vi "TDC_DAQV31_Paralled_muon.vi"(7 "address":string[](array[string])=["192.168.10.20"], 8 "error in (no error)":errorcluster, 9 "stop":bool, 10 "save data":bool=TRUE, 11 "SMA mode":bool=TRUE) -> (0 "error out 3":errorcluster, 2 "csv path":path=path "G:/tdc/2017/data/test_20250313_082908.csv", 3 "rate":dbl)   [LabVIEW 2017]
uses:
  gloabal.vi
  <vilib>/Utility/file.llb/Write Delimited Spreadsheet (DBL).vi
  <vilib>/Utility/file.llb/Write Delimited Spreadsheet (I64).vi
panel:
  out "x .and. y?":u64
  out "pmt trigger rate":u32[](array[numeric])
  out "event":u32[](array[numeric])
  in  "calib_file":path=path "G:/tdc/2017/data/test_20250313_032748_codeDensity.csv" caption="文件路径 （空时为对话框）"
  in  "use_calib_file":bool
  out "cal 3":u32[](graph)=[0, 0, 0, 0, 0, 0, 0, 0, 0, 0, 0, 0, 0, 0, 0, 0, 0, 0, 0, 0, 0, 0, 0, 0, 0, 0, 0, 0, 0, 0, 0, 0, 0, 0, 0, 0, 0, 0, 0, 0, 0, 0, 0, 0, 0, 0, 0, 0, 0, 0, 0, 0, 0, 0, 0, 0, 0, 0, 0, 0, 0, 0, 0, 0, 0, 0, 0, 0, 0, 0, 0, 0, 0, 0, 0, 0, 0, 0, 0, 0, 0, 0, 0, 0, 0, 0, 0, 0, 0, 0, 0, 0, 0, 0, 0, 0, 0, 0, 0, 0, 0, 0, 0, 0, 0, 0, 0, 0, 0, 0, 0, 0, 0, 0, 0, 0, 0, 0, 0, 0, 0, 0, 0, 0, 0, 0, 0, 0, 0, 0, 0, 0, 0, 0, 0, 0, 0, 0, 0, 0, 0, 0, 0, 0, 0, 0, 0, 0, 0, 0, 0, 0, 0, 0, 0, 0, 0, 0, 0, 0, 0, 0, 0, 0, 0, 15, 3, 1, 14, 3, 31, 20, 16, 6, 1, 18, 12, 4, 29, 10, 8, 29, 2, 14, 4, 25, 7, 24, 4, 0, 1, 5, 8, 18, 22, 0, 4, 5, 0, 12, 9, 9, 20, 21, 4, 10, 13, 5, 21, 13, 14, 2, 6, 13, 1, 3, 5, 10, 20, 2, 3, 4, 3, 4, 2, 20, 13, 2, 5, 1, 3, 12, 4, 1, 14, 7, 5, 4, 1, 10, 2, 21, 14, 2, 5, 10, 4, 0, 11, 19, 6, 4, 1, 37, 1, 4, 2, 1, 10, 13, 4, 8, 10, 6, 9, 2, 0, 6, 8, 12, 3, 21, 5, 7, 8, 2, 3, 7, 17, 6, 5, 6, 4, 6, 0, 2, 1, 3, 10, 33, 7, 2, 6, 3, 7, 3, 2, 0, 12, 10, 11, 13, 13, 7, 3, 9, 6, 16, 0, 13, 5, 6, 3, 0, 5, 5, 7, 1, 10, 7, 13, 14, 5, 1, 12, 7, 1, 10, 2, 1, 14, 18, 13, 11, 4, 6, 9, 22, 11, 9, 2, 2, 8, 14, 4, 4, 6, 12, 13, 3, 9, 5, 5, 1, 5, 11, 18, 3, 0, 5, 4, 6, 7, 6, 1, 13, 5, 1, 2, 2, 1, 4, 12, 7, 3, 2, 3, 9, 11, 1, 20, 3, 4, 5, 5, 3, 5, 8, 5, 3, 26, 14, 6, 1, 3, 12, 12, 4, 23, 10, 3, 4, 4, 10, 3, 5, 4, 2, 14, 5, 15, 20, 1, 5, 1, 20, 6, 1, 3, 13, 21, 12, 7, 4, 1, 5, 30, 11, 2, 4, 0, 12, 7, 10, 3, 2, 25, 6, 1, 3, 6, 3, 8, 37, 4, 6, 2, 2, 4, 3, 5, 6, 13, 6, 9, 22, 1, 3, 7, 7, 4, 8, 33, 2, 1, 15, 3, 8, 23, 21, 2, 2, 27, 13, 3, 5, 10, 4, 18, 5, 5, 8, 0, 1, 8, 12, 4, 3, 0, 4, 8, 4, 7, 4, 2, 11, 13, 3, 0, 7, 5, 3, 4, 8, 4, 20, 2, 13, 4, 8, 6, 17, 4, 2, 1, 15, 2, 15, 5, 19, 0, 4, 15, 4, 16, 11, 1, 16, 4, 6, 6, 5, 7, 3, 9, 15, 3, 6, 3, 13, 5, 7, 3, 27, 2, 0, 21, 1, 4, 1, 4, 5, 3, 10, 7, 3, 6, 4, 18, 21, 7, 6, 7, 7, 12, 6, 9, 8, 11, 12, 13, 2, 2, 5, 4, 7, 52, 3, 5, 8, 7, 10, 4, 4, 6, 5, 18, 0, 3, 6, 1, 9, 5, 19, 13, 24, 12, 4, 4, 15, 6, 41, 3, 8, 5, 17, 26, 8, 7, 20, 2, 5, 12, 10, 10, 12, 9, 17, 6, 3, 1, 5, 3, 7, 8, 4, 10, 5, 10, 7, 1, 2, 14, 7, 25, 3, 0, 0, 0, 5, 21, 8, 14, 4, 10, 2, 3, 2, 4, 8, 12, 3, 6, 8, 3, 4, 3, 20, 5, 6, 7, 8, 11, 2, 8, 6, 5, 15, 17, 10, 10, 3, 3, 9, 18, 7, 7, 3, 5, 5, 5, 2, 2, 2, 4, 1, 0, 42, 3, 14, 4, 3, 5, 2, 7, 4, 2, 7, 5, 22, 4, 3, 17, 3, 5, 8, 19, 7, 5, 0, 3, 4, 10, 1, 8, 2, 2, 13, 23, 4, 9, 5, 0, 0, 0, 27, 2, 16, 11, 15, 3, 0, 18, 2, 8, 29, 19, 6, 7, 2, 6, 12, 1, 13, 2, 7, 5, 11, 8, 5, 6, 6, 19, 2, 4, 0, 7, 22, 13, 3, 7, 3, 8, 11, 0, 3, 26, 6, 5, 5, 6, 4, 10, 17, 16, 4, 3, 4, 3, 4, 21, 8, 10, 10, 7, 0, 9, 9, 2, 10, 10, 2, 9, 9, 4, 14, 5, 5, 4, 18, 6, 3, 0, 4, 1, 20, 2, 33, 4, 1, 2, 1, 20, 6, 3, 11, 10, 2, 1, 13, 9, 6, 1, 0, 0, 0, 0, 0, 0, 0, 0, 0, 0, 0, 0, 0, 0, 0, 0, 0, 0, 0, 0, 0, 0, 0, 0, 0, 0, 0, 0, 0, 0, 0, 0, 0, 0, 0, 0, 0, 0, 0, 0, 0, 0, 0, 0, 0, 0, 0, 0, 0, 0, 0, 0, 0, 0, 0, 0, 0, 0, 0, 0, 0, 0, 0, 0, 0, 0, 0, 0, 0, 0, 0, 0, 0, 0, 0, 0, 0, 0, 0, 0, 0, 0, 0, 0, 0, 0, 0, 0, 0, 0, 0, 0, 0, 0, 0, 0, 0, 0, 0, 0, 0, 0, 0, 0, 0, 0, 0, 0, 0, 0, 0, 0, 0, 0, 0, 0, 0, 0, 0, 0, 0, 0, 0, 0, 0, 0, 0, 0, 0, 0, 0, 0, 0, 0, 0, 0, 0, 0, 0, 0, 0, 0, 0, 0, 0, 0, 0, 0, 0, 0, 0, 0, 0, 0, 0, 0, 0, 0, 0, 0, 0, 0, 0, 0, 0, 0, 0, 0, 0, 0, 0, 0, 0, 0, 0, 0, 0, 0, 0, 0, 0, 0, 0, 0, 0, 0, 0, 0, 0, 0, 0, 0, 0, 0, 0, 0, 0, 0, 0, 0, 0, 0, 0, 0, 0, 0, 0, 0, 0, 0, 0, 0, 0, 0, 0, 0, 0, 0, 0, 0, 0, 0, 0, 0, 0, 0, 0, 0, 0, 0, 0, 0, 0, 0, 0, 0, 0, 0, 0, 0, 0, 0, 0, 0, 0, 0, 0, 0, 0, 0, 0, 0, 0, 0, 0, 0, 0, 0, 0, 0, 0, 0, 0, 0, 0, 0, 0, 0, 0, 0, 0, 0, 0, 0, 0, 0, 0, 0, 0, 0, 0, 0, 0, 0, 0, 0, 0, 0, 0, 0, 0, 0, 0, 0, 0, 0, 0, 0, 0, 0, 0, 0, 0, 0, 0, 0, 0, 0, 0, 0, 0, 0, 0, 0, 0, 0, 0, 0, 0, 0, 0, 0, 0, 0, 0, 0, 0, 0, 0, 0, 0, 0, 0, 0, 0, 0, 0, 0, 0, 0, 0, 0, 0, 0, 0, 0, 0, 0, 0, 0, 0, 0, 0, 0, 0, 0, 0, 0, 0, 0, 0, 0, 0, 0, 0, 0, 0, 0, 0, 0, 0, 0, 0, 0, 0, 0, 0, 0, 0, 0, 0, 0, 0, 0, 0, 0, 0, 0, 0, 0, 0, 0, 0, 0, 0, 0, 0, 0, 0, 0, 0, 0, 0, 0, 0, 0, 0, 0, 0, 0, 0, 0, 0, 0, 0, 0, 0, 0, 0, 0, 0, 0, 0, 0, 0, 0, 0, 0, 0, 0, 0, 0, 0, 0, 0, 0, 0, 0, 0, 0, 0, 0, 0, 0, 0, 0, 0, 0, 0, 0, 0, 0, 0, 0, 0, 0, 0, 0, 0, 0, 0, 0, 0, 0, 0, 0, 0, 0, 0, 0, 0, 0, 0, 0, 0, 0, 0, 0, 0, 0, 0, 0, 0, 0, 0, 0, 0, 0, 0, 0, 0, 0, 0, 0, 0, 0, 0, 0, 0, 0, 0, 0, 0, 0, 0, 0, 0, 0, 0, 0, 0, 0, 0, 0, 0, 0, 0, 0, 0, 0, 0, 0, 0, 0, 0, 0, 0, 0, 0, 0, 0, 0, 0, 0, 0, 0, 0, 0, 0, 0, 0, 0, 0, 0, 0, 0, 0, 0, 0, 0, 0, 0, 0, 0, 0, 0, 0, 0, 0, 0, 0, 0, 0, 0, 0, 0, 0, 0, 0, 0, 0, 0, 0, 0, 0, 0, 0, 0, 0, 0, 0, 0, 0, 0, 0, 0, 0, 0, 0, 0, 0, 0, 0, 0, 0, 0, 0, 0, 0, 0, 0, 0, 0, 0, 0, 0, 0, 0, 0, 0, 0, 0, 0, 0, 0, 0, 0, 0, 0, 0, 0, 0, 0, 0, 0, 0, 0, 0, 0, 0, 0, 0, 0, 0, 0, 0, 0, 0, 0, 0, 0, 0, 0, 0, 0, 0, 0, 0, 0, 0, 0, 0, 0, 0, 0, 0, 0, 0, 0, 0, 0, 0, 0, 0, 0, 0, 0, 0, 0, 0, 0, 0, 0, 0, 0, 0, 0, 0, 0, 0, 0, 0, 0, 0, 0, 0, 0, 0, 0, 0, 0, 0, 0, 0, 0, 0, 0, 0, 0, 0, 0, 0, 0, 0, 0, 0, 0, 0, 0, 0, 0, 0, 0, 0, 0, 0, 0, 0, 0, 0, 0, 0, 0, 0, 0, 0, 0, 0, 0, 0, 0, 0, 0, 0, 0, 0, 0, 0, 0, 0, 0, 0, 0, 0, 0, 0, 0, 0, 0, 0, 0, 0, 0, 0, 0, 0, 0, 0, 0, 0, 0, 0, 0, 0, 0, 0, 0, 0, 0, 0, 0, 0, 0, 0, 0, 0, 0, 0, 0, 0, 0, 0, 0, 0, 0, 0, 0, 0, 0, 0, 0, 0, 0, 0, 0, 0, 0, 0, 0, 0, 0, 0, 0, 0, 0, 0, 0, 0, 0, 0, 0, 0, 0, 0, 0, 0, 0, 0, 0, 0, 0, 0, 0, 0, 0, 0, 0, 0, 0, 0, 0, 0, 0, 0, 0, 0, 0, 0, 0, 0, 0, 0, 0, 0, 0, 0, 0, 0, 0, 0, 0, 0, 0, 0, 0, 0, 0, 0, 0, 0, 0, 0, 0, 0, 0, 0, 0, 0, 0, 0, 0, 0, 0, 0, 0, 0, 0, 0, 0, 0, 0, 0, 0, 0, 0, 0, 0, 0, 0, 0, 0, 0, 0, 0, 0, 0, 0, 0, 0, 0, 0, 0, 0, 0, 0, 0, 0, 0, 0, 0, 0, 0, 0, 0, 0, 0, 0, 0, 0, 0, 0, 0, 0, 0, 0, 0, 0, 0, 0, 0, 0, 0, 0, 0, 0, 0, 0, 0, 0, 0, 0, 0, 0, 0, 0, 0, 0, 0, 0, 0, 0, 0, 0, 0, 0, 0, 0, 0, 0, 0, 0, 0, 0, 0, 0, 0, 0, 0, 0, 0, 0, 0, 0, 0, 0, 0, 0, 0, 0, 0, 0, 0, 0, 0, 0, 0, 0, 0, 0, 0, 0, 0, 0, 0, 0, 0, 0, 0, 0, 0, 0, 0, 0, 0, 0, 0, 0, 0, 0, 0, 0, 0, 0, 0, 0, 0, 0, 0, 0, 0, 0, 0, 0, 0, 0, 0, 0, 0, 0, 0, 0, 0, 0, 0, 0, 0, 0, 0, 0, 0, 0, 0, 0, 0, 0, 0, 0, 0, 0, 0, 0, 0, 0, 0, 0, 0, 0, 0, 0, 0, 0, 0, 0, 0, 0, 0, 0, 0, 0, 0, 0, 0, 0, 0, 0, 0, 0, 0, 0, 0, 0, 0, 0, 0, 0, 0, 0, 0, 0, 0, 0, 0, 0, 0, 0, 0, 0, 0, 0, 0, 0, 0, 0, 0, 0, 0, 0, 0, 0, 0, 0, 0, 0, 0, 0, 0, 0, 0, 0, 0, 0, 0, 0, 0, 0, 0, 0, 0, 0, 0, 0, 0, 0, 0, 0, 0, 0, 0, 0, 0, 0, 0, 0, 0, 0, 0, 0, 0, 0, 0, 0, 0, 0, 0, 0, 0, 0, 0, 0, 0, 0, 0, 0, 0, 0, 0, 0, 0, 0, 0, 0, 0, 0, 0, 0, 0, 0, 0, 0, 0, 0, 0, 0, 0, 0, 0, 0, 0, 0, 0, 0, 0, 0, 0, 0, 0, 0, 0, 0, 0, 0, 0, 0, 0, 0, 0, 0, 0, 0, 0, 0, 0, 0, 0, 0, 0, 0, 0, 0, 0, 0, 0, 0, 0, 0]
  out "second stamp":u64=57608
  in  "coarse counter width":u16(ring) items=["29", "48"]
  out "name (unnamed)":string
  out "error out 5":errorcluster
  in  "timeout":dbl=30000.0
  out "DAC":dbl=8094.0
  out "Out":u8=3 format="%.0x"
  out "fine 4":u64=133527214080 format="%x"
  out "coarse":u64=65198835 format="%x"
  in  "gps":bool
  out "Year":string="2025"
  in  "factor":i32=128
  in  "displayCR":bool=TRUE
  in  "Counter Setting":dbl=100000.0 format="%#_13g"
  in  "replace dat":bool
  in  "append csv":bool=TRUE
  out "element":string
  out "fine":u64=593 format="%x"
  in  "UDP Config":bool=TRUE
  in  "data  path":path=path "G:/tdc/2017/data"
  out "cal 2":u64[](graph)
  in  "Thresholds (mV)":dbl[](array[numeric])=[580.0, 580.0, 580.0, 580.0, 600.0, 600.0, 600.0, 600.0, 580.0, 580.0, 600.0, 600.0, 600.0, 600.0, 600.0, 600.0, 580.0, 580.0, 600.0, 600.0, 600.0, 600.0, 600.0, 600.0, 580.0, 580.0, 600.0, 600.0, 600.0, 600.0, 600.0, 600.0, 600.0, 600.0, 600.0, 600.0, 600.0, 600.0, 600.0, 600.0, 600.0, 600.0, 600.0, 600.0, 600.0, 600.0, 600.0, 600.0, 600.0, 600.0, 600.0, 600.0, 600.0, 600.0, 600.0, 600.0, 600.0, 600.0, 600.0, 600.0, 600.0, 600.0, 600.0, 600.0]
  out "error out 2":errorcluster
  in  "display":bool=TRUE
  in  "Thresholds":dbl=-0.03
  in  "one key for threshold":bool=TRUE
  in  "RST":bool
  in  "通道数量":i32=128
  out "Cal Table":u32[](array[numeric])
  in  "channel for cal":i32=3
  out "channel number":u64
  out "Calibration Counter":i32=100000
  out "Event index":i32=97959
  out "cal":i64[](graph)
  out "error out":errorcluster
  out "appended path":path=path "G:/tdc/2017/data/test_20250313_082908.dat"
  in  "filename":string="test"
  in  "Events":i32=110000 min=1
  in  "timeout (ms)":i32=10000
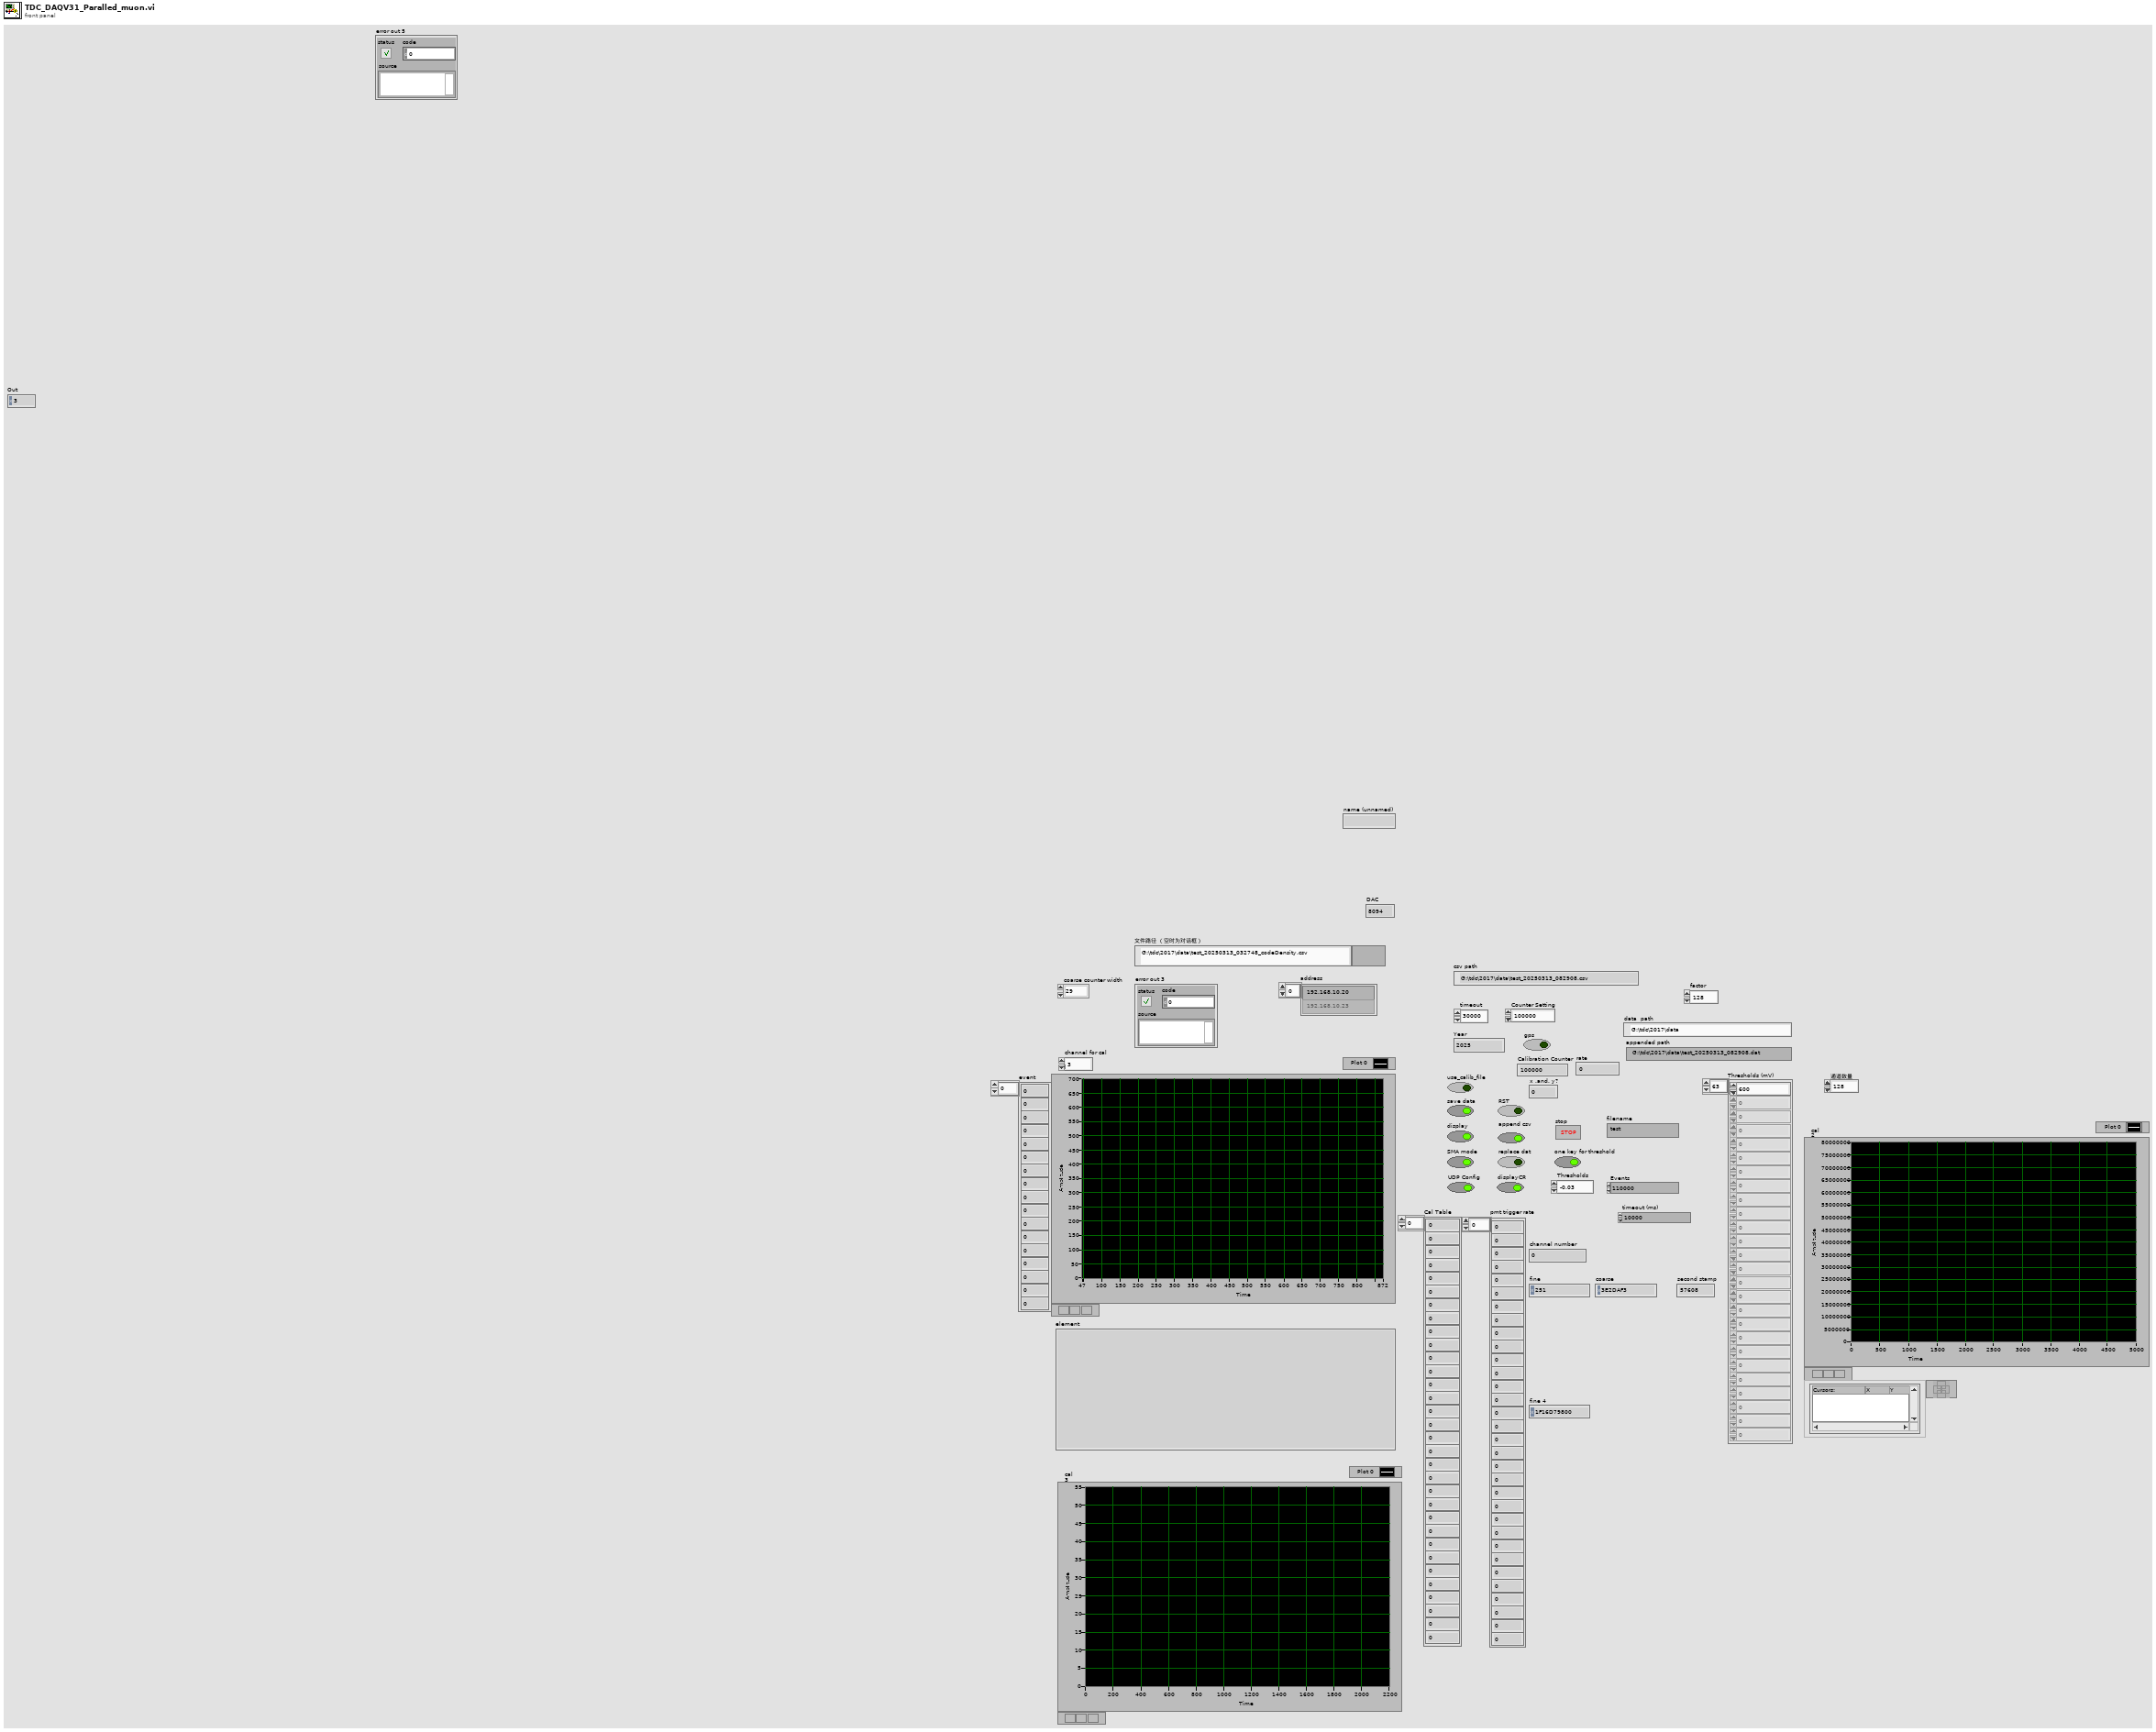
[diagram p1: front panel]
types:
  T1 = enum16{"open", "replace", "create", "open or create", "replace or create", "replace or create with confirmation"}
  T2 = enum16{"big-endian, network order", "native, host order", "little-endian"}
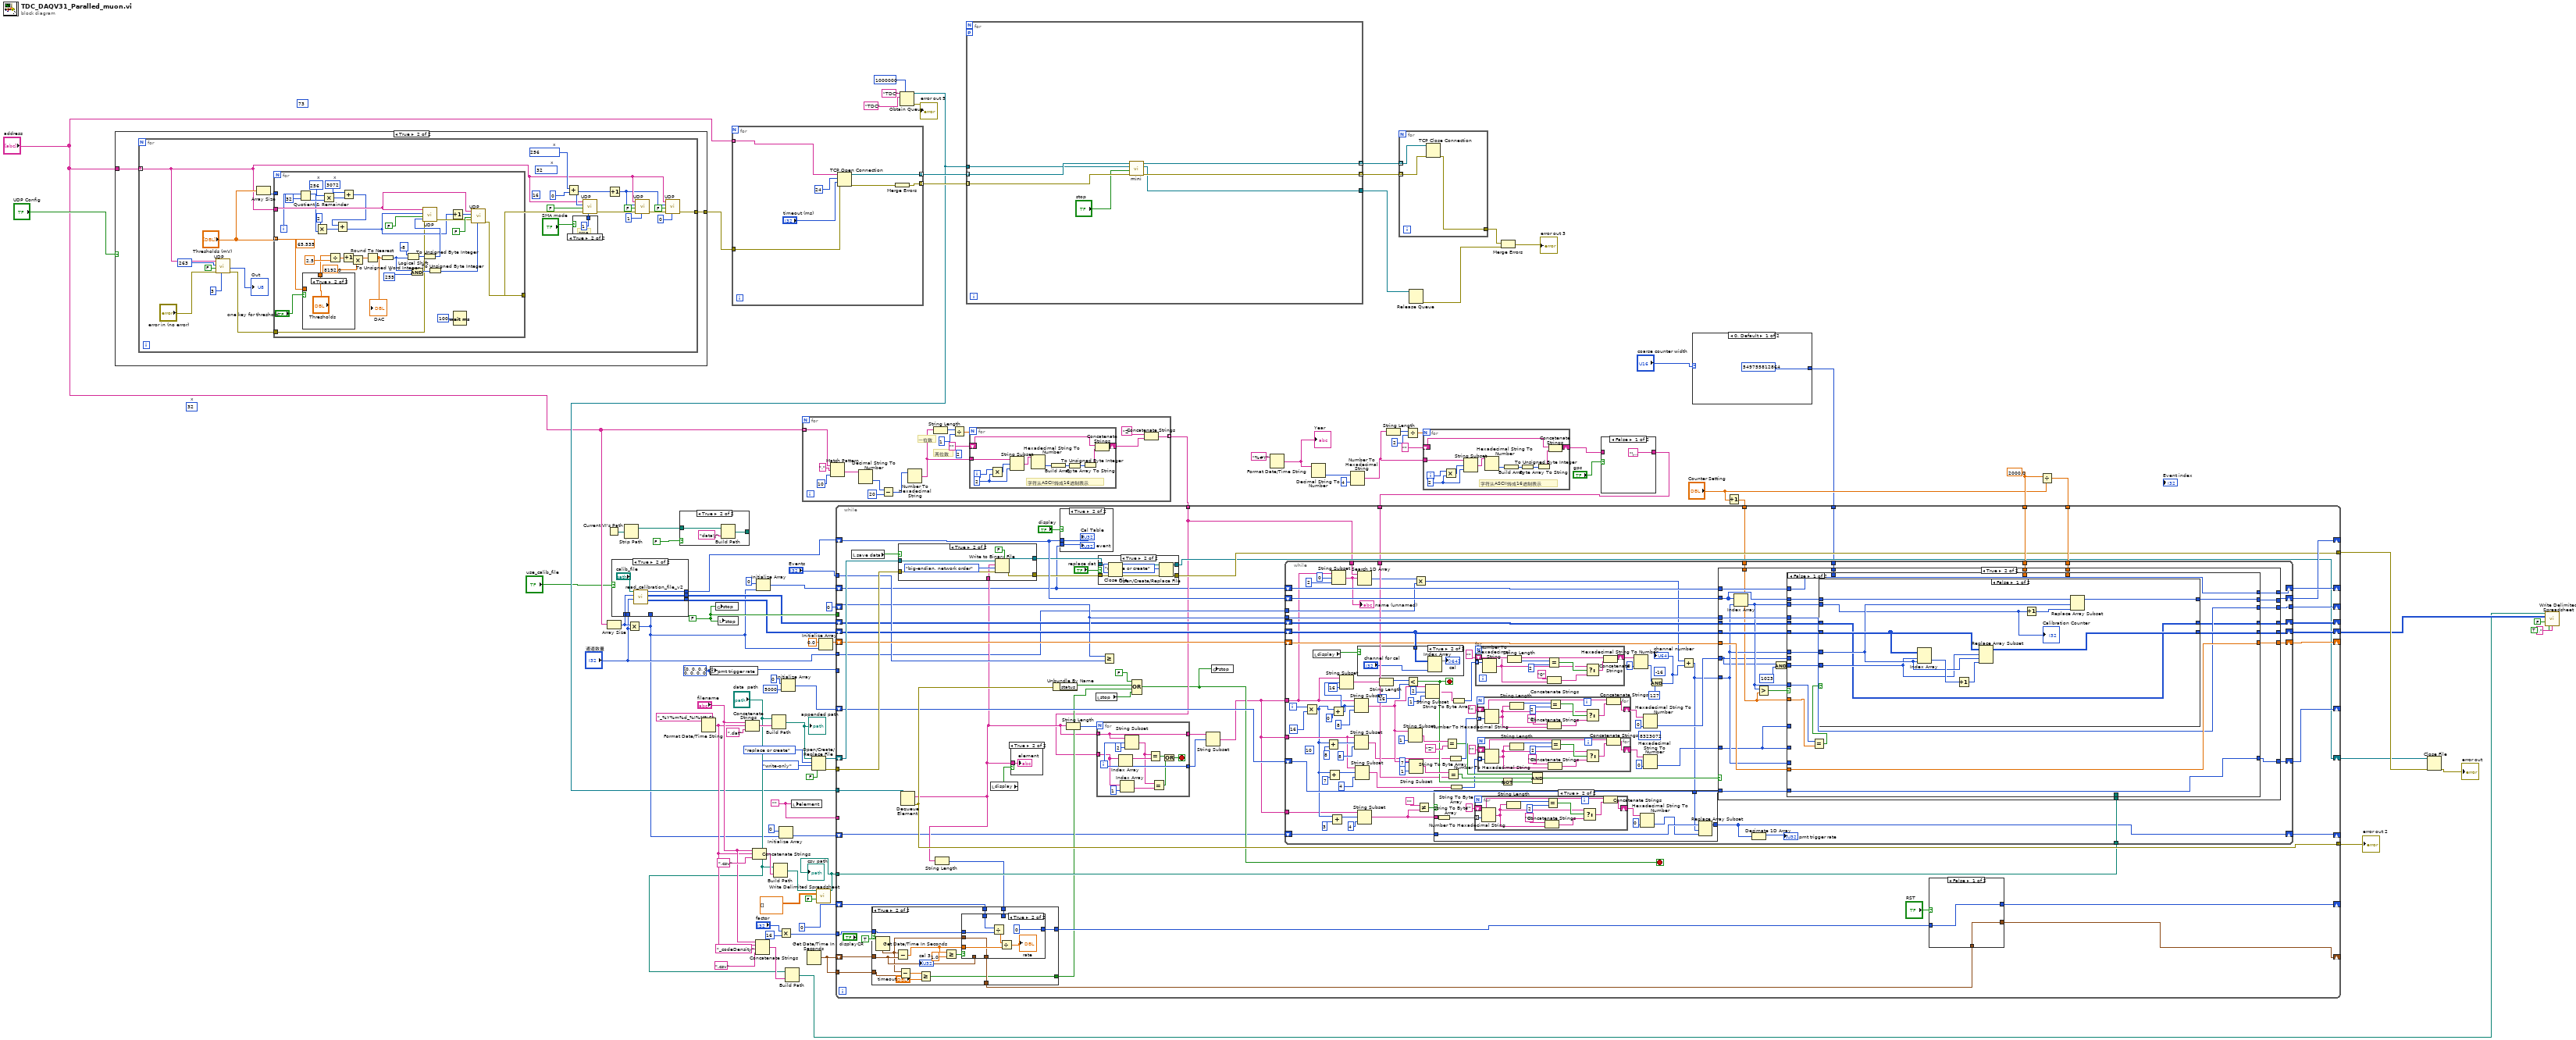
[diagram p0: block diagram]
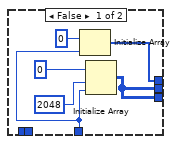
[diagram p2: hidden frame]
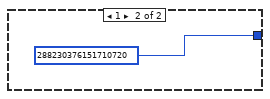
[diagram p3: hidden frame]
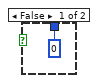
[diagram p6: hidden frame]
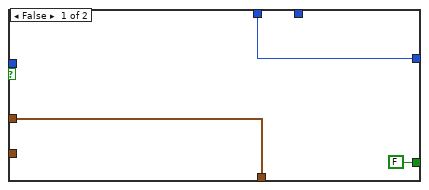
[diagram p12: hidden frame]
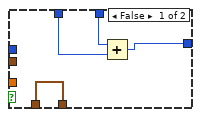
[diagram p13: hidden frame]
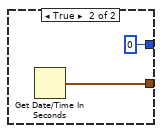
[diagram p15: hidden frame]
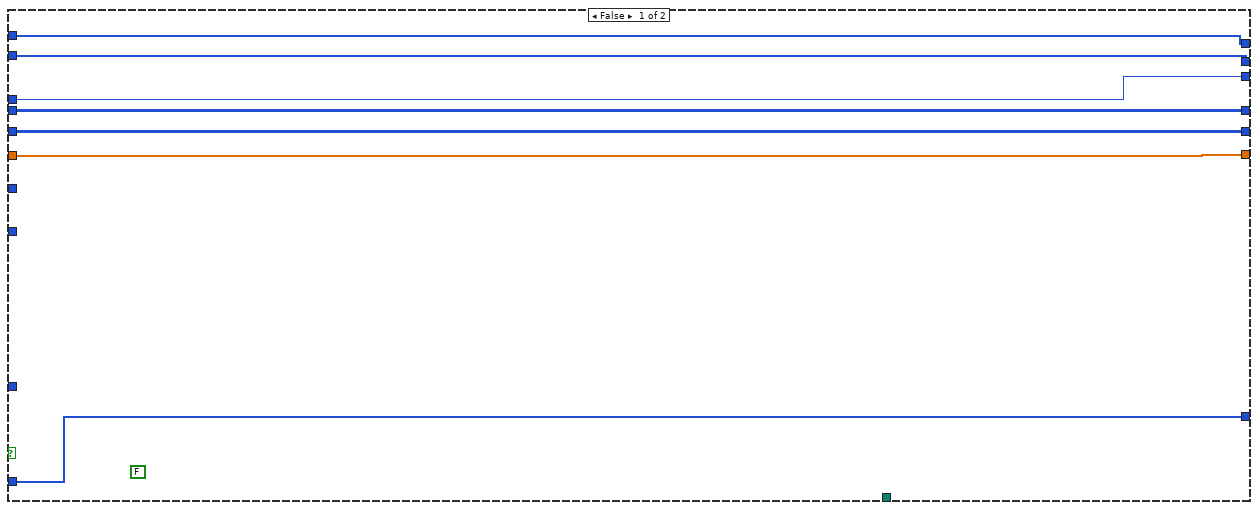
[diagram p18: hidden frame]
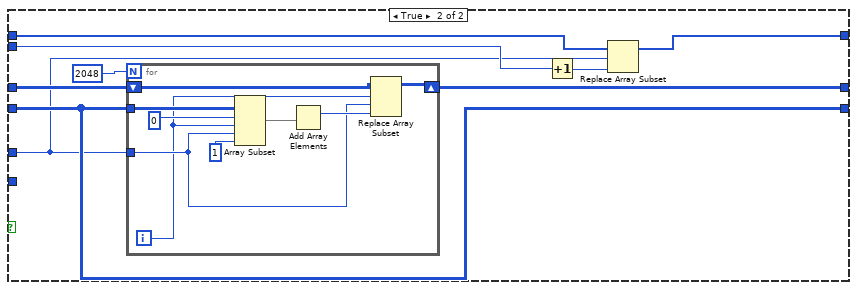
[diagram p19: hidden frame]
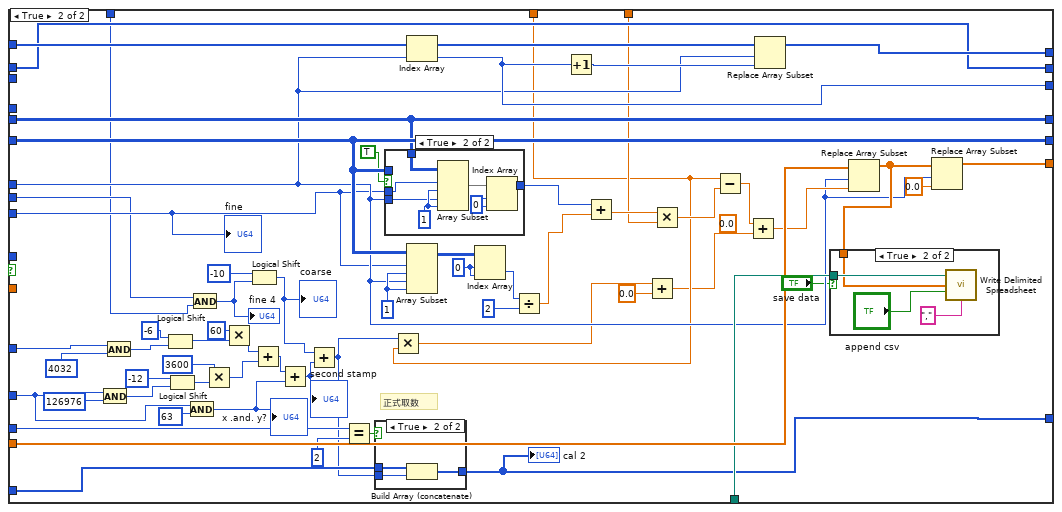
[diagram p20: hidden frame]
diagram:
  w1 = ""
  w2 = u32[] [0, 0, 0, 0, 0, 0, 0, 0, 0, 0, 0, 0, 0, 0, 0, 0, 0, 0, 0, 0, 0, 0, 0, 0, 0, 0, 0, 0, 0, 0, 0, 0, 0, 0, 0, 0, 0, 0, 0, 0, 0, 0, 0, 0, 0, 0, 0, 0, 0, 0, 0, 0, 0, 0, 0, 0, 0, 0, 0, 0, 0, 0, 0, 0] ("pmt trigger rate")
  (unwired) u32 73 ("Address")
  w53 = 2000.0 ("x")
  (unwired) u16 32  # x
  w15 = FALSE ("stop")
  n1 = case shown="True" "UDP Config" {
    tunnel: "address" -> [_ w95]
    tunnel: [_ w96] -> w20
    frame False {
    }
    frame True {
      n2 = for {
        tunnel: [w101] -> w96
        tunnel: w95 -> [w99] mode=indexing
        (unwired) u16 32  # x
        (unwired) u32 16 ("Address")
        w113 = u16 256  # x
        n3 = call "UDP.vi"("In"=u8 3, "error in (no error)"="error in (no error)", "Read (TRUE)"=FALSE, "Address"=u32 263, "IP address"=w99) -> ("error out"=w107:errorcluster, "Out"=→"Out":u8)  [unwired: 3 in, 1 out]
        n4 = Array Size(array="Thresholds (mV)") -> (size(s)=w116:i32)
        n5 = for {
          tunnel: w99 -> [w152]
          tunnel: "Thresholds (mV)" -> [w139] mode=indexing
          tunnel: [w142] -> w119
          tunnel: w116 -> [_]
          tunnel: w107 -> [w126]
          i -> [w134]
          (unwired) 65.535 ("y")
          w135 = u16 3072  # x
          w136 = u16 256  # x
          w148 = u16 255  # x
          n6 = Quotient & Remainder(x=w134, y=32) -> (x-y*floor(x/y)=w128:i32, floor(x/y)=w137:i32)
          n7 = case shown="True" "one key for threshold" {
            tunnel: [w158 "Thresholds"] -> w140
            tunnel: w139 -> [w158 _]
            frame False {
            }
            frame True {
            }
          }
          n8 = Multiply(x=2, y=w128) -> (x*y=w129:i32)
          n9 = Multiply(x=w136, y=w137) -> (x*y=w131:i32)
          n10 = Divide(x=w140, y=2.5) -> (x/y=w155:dbl)
          n11 = Increment(x=w155) -> (x+1=w125:dbl)
          n12 = Add(x=w135, y=w131) -> (x+y=w130:i32)
          n13 = Add(x=w130, y=w129) -> (x+y=w133:i32)
          n14 = Multiply(x=w125, y=8192.0) -> (x*y=w124:dbl)
          n15 = Round To Nearest(number=w124) -> (nearest integer value=w153:dbl)
          "DAC" <- w153
          n16 = To Unsigned Word Integer(number=w153) -> (unsigned 16bit integer=w144:u16)
          n17 = Logical Shift(y=i16 -8, x=w144) -> (x << y=w150:u16)
          n18 = And(x=w144, y=w148) -> (x .and. y?=w147:u16)
          n19 = To Unsigned Byte Integer(number=w150) -> (unsigned 8bit integer=w149:u8)
          n20 = call "UDP.vi"("In"=w149, "error in (no error)"=w126, "Read (TRUE)"=FALSE, "Address"=w133, "IP address"=w152) -> ("error out"=w143:errorcluster)  [unwired: 3 in, 2 out]
          n21 = To Unsigned Byte Integer(number=w147) -> (unsigned 8bit integer=w146:u8)
          n22 = Increment(x=w133) -> (x+1=w132:i32)
          n23 = Wait (ms)(milliseconds to wait=u32 100) -> ()  [unwired: 1 out]
          n24 = call "UDP.vi"("In"=w146, "error in (no error)"=w143, "Read (TRUE)"=FALSE, "Address"=w132, "IP address"=w152) -> ("error out"=w142:errorcluster)  [unwired: 3 in, 2 out]
        }
        n25 = Add(x=w113, y=u32 0 ("Address")) -> (x+y=w105:u32)
        n26 = case shown="True" "SMA mode" {
          tunnel: [u8 0 ("In") u8 1 ("In")] -> w118
          frame False {
          }
          frame True {
            # "sma"
          }
        }
        n27 = call "UDP.vi"("In"=w118, "error in (no error)"=w119, "Read (TRUE)"=FALSE, "Address"=w105, "IP address"=w99) -> ("error out"=w106:errorcluster)  [unwired: 3 in, 2 out]
        n28 = Increment(x=w105) -> (x+1=w98:u32)
        n29 = call "UDP.vi"("In"=u8 1, "error in (no error)"=w106, "Read (TRUE)"=FALSE, "Address"=w98, "IP address"=w99) -> ("error out"=w102:errorcluster)  [unwired: 3 in, 2 out]
        n30 = call "UDP.vi"("In"=u8 0, "error in (no error)"=w102, "Read (TRUE)"=FALSE, "Address"=w98, "IP address"=w99) -> ("error out"=w101:errorcluster)  [unwired: 3 in, 2 out]
      }
    }
  }
  n31 = Current VI's Path() -> (path=w89:path)
  n32 = Array Size(array="address") -> (size(s)=w7:i32)
  n33 = Strip Path(path=w89) -> (stripped path=w88:path)  [unwired: 1 out]
  n34 = Multiply(x=w7, y="通道数量") -> (x*y=w4:i32)
  n35 = case shown="True" "use_calib_file" {
    tunnel: w4 -> [w163 _]
    tunnel: [w160 w171] -> w10
    tunnel: [w160 w170] -> w9
    tunnel: [w161 w169] -> w8
    tunnel: w7 -> [_ w168]
    tunnel: "通道数量" -> [_ w167]
    frame False {
      n36 = Initialize Array(u32 0 ("element"), w163) -> (w161:u32[])
      n37 = Initialize Array(u32 0 ("element"), 2048 ("dimension size"), w163) -> (w160:u32[][])
    }
    frame True {
      n38 = call "read_calibration_file_v2.vi"("通道数量"=w167, "板子数量"=w168, "file path (dialog if empty)"="calib_file") -> ("code_density"=w171:i64[][], "accumulation"=w170:u32[][], "Cal Table"=w169:u32[])  [unwired: 5 in, 1 out]
    }
  }
  n39 = case shown="True" FALSE {
    tunnel: w88 -> [w172 w174]
    tunnel: [w172 w173] -> _
    frame False {
    }
    frame True {
      n40 = Build Path(base path=w174, name or relative path="data\\") -> (appended path=w173:path)
    }
  }
  n41 = Format Date/Time String(time format string (%c)="_%Y%m%d_%I%M%S") -> (date/time string=w70:string)  [unwired: 2 in]
  n42 = local write "pmt trigger rate"(w2) -> ()
  n43 = global write "gloabal.vi" "stop"(w15) -> ()
  n44 = local write "stop"(w15) -> ()
  n45 = for {
    tunnel: "address" -> [w181] mode=indexing
    tunnel: [w180] -> w30 mode=indexing
    tunnel: [w178] -> w29 mode=indexing
    tunnel: w20 -> [w177]
    n46 = TCP Open Connection(address=w181, remote port or service name=u16 24 ("port"), timeout ms (60000)="timeout (ms)", error in (no error)=w177) -> (connection ID=w180:refnum<k5>, error out=w179:errorcluster)  [unwired: 1 in]
    n47 = Merge Errors(w179) -> (w178:errorcluster)
  }
  n48 = Concatenate Strings("filename", w70, ".dat") -> (w87:string)
  n49 = Concatenate Strings("filename", w70, ".csv") -> (w77:string)
  n50 = Concatenate Strings("filename", w70, "_codeDensity" ("string"), ".csv") -> (w67:string)
  n51 = Initialize Array(u32 0 ("element"), w4) -> (w76:u32[])
  n52 = Build Path(base path="data  path", name or relative path=w87) -> (appended path=w86:path)
  "appended path" <- w86
  n53 = Build Path(base path="data  path", name or relative path=w77) -> (appended path=w74:path)
  n54 = Initialize Array(u32 0 ("element"), w4) -> (w3:u32[])
  n55 = Multiply(x="factor", y=16) -> (x*y=w46:i32)
  n56 = Initialize Array(u32 0 ("element"), 5000 ("dimension size")) -> (w58:u32[])
  n57 = Build Path(base path="data  path", name or relative path=w67) -> (appended path=w64:path)
  n58 = local write "element"(w1) -> ()
  n59 = for {
    tunnel: [w184] -> w32 mode=indexing
    tunnel: "address" -> [w183] mode=indexing
    (unwired) 2 ("y")
    # "一位数"
    # "两位数"
    n60 = Match Pattern(string=w183, regular expression="." ("search string"), offset (0)=10) -> (after substring=w190:string)  [unwired: 3 out]
    n61 = Decimal String To Number(string=w190) -> (number=w187:i32)  [unwired: 2 in, 1 out]
    n62 = Subtract(x=w187, y=20) -> (x-y=w186:i32)
    n63 = Number To Hexadecimal String(2:w186) -> (0:w189:string)  [unwired: 1 in]
    n64 = String Length(string=w189) -> (length=w195:i32)
    n65 = Divide(x=w195, y=1) -> (x/y=w196:dbl)
    n66 = for {
      N: w196 -> [_]
      shift-right: [w208] -> w185
      shift-left: "" ("format string") -> [w207]
      tunnel: w189 -> [w198]
      i -> [w206]
      w200 = 2 ("y")
      # "字符从ASCII转成16进制表示"
      n67 = Multiply(x=w206, y=w200) -> (x*y=w199:i32)
      n68 = String Subset(string=w198, offset (0)=w199, length (rest)=w200) -> (substring=w201:string)
      n69 = Hexadecimal String To Number(string=w201) -> (number=w205:u32)  [unwired: 2 in, 1 out]
      n70 = Build Array(w205) -> (w204:u32[])
      n71 = To Unsigned Byte Integer(number=w204) -> (unsigned 8bit integer=w203:u8[])
      n72 = Byte Array To String(unsigned byte array=w203) -> (string=w202:string)
      n73 = Concatenate Strings(w207, w202) -> (w208:string)
    }
    n74 = Concatenate Strings("Z", w185) -> (w184:string)
  }
  n75 = Get Date/Time In Seconds() -> (seconds since 1Jan1904=w31:timestamp)
  n76 = Open/Create/Replace File(file path (use dialog)=w86, operation (0:open)=T1."replace or create", access (0:read/write)=enum16{"read/write", "read-only", "write-only"}."write-only", disable buffering (F)=FALSE) -> (refnum out=w91:refnum<file>, error out=w90:errorcluster)  [unwired: 2 in, 1 out]
  n77 = call-poly <vilib>:"Write Delimited Spreadsheet.vi"("file path (dialog if empty)"=w74, "2D data"=dbl[][] [], "append to file? (new file:F)"=FALSE) -> ("new file path (Not A Path if cancelled)"=w14:path)  [unwired: 11 in, 1 out]
  "csv path" <- w14
  n78 = Initialize Array(0.0, w4) -> (w60:dbl[])
  n79 = Obtain Queue(max queue size (-1, unlimited)=1000000, name (unnamed)="TDC", element data type="TDC" ("name (unnamed)")) -> (queue out=w21:refnum<queue>, error out=→"error out 5":errorcluster)  [unwired: 2 in, 1 out]
  n80 = for {
    tunnel: w30 -> [w215] mode=indexing
    tunnel: w29 -> [w214] mode=indexing
    tunnel: [w213] -> w28 mode=indexing
    tunnel: [w212] -> w27 mode=indexing
    workers-P: _ -> [_]
    tunnel: w21 -> [w211]
    tunnel: [w210] -> w22
    n81 = call "mini.vi"("error in (no error)"=w214, "stop"="stop", "queue out 2"=w211, "connection ID 2"=w215) -> ("error out 3"=w212:errorcluster, "queue out"=w210:refnum<queue>, "connection ID"=w213:refnum<k5>)  [unwired: 5 in]
  }
  n82 = Format Date/Time String(time format string (%c)="%#Y") -> (date/time string=w43:string)  [unwired: 2 in]
  "Year" <- w43
  n83 = Decimal String To Number(string=w43) -> (number=w42:i32)  [unwired: 2 in, 1 out]
  n84 = Number To Hexadecimal String(1:i16 4 ("width (-)"), 2:w42) -> (0:w36:string)
  n85 = String Length(string=w36) -> (length=w38:i32)
  n86 = for {
    tunnel: w28 -> [w218] mode=indexing
    tunnel: w27 -> [w217] mode=indexing
    tunnel: [w216] -> w19
    n87 = TCP Close Connection(connection ID=w218, error in (no error)=w217) -> (error out=w216:errorcluster)  [unwired: 1 in, 1 out]
  }
  n88 = Divide(x=w38, y=2) -> (x/y=w39:dbl)
  n89 = Release Queue(queue=w22) -> (error out=w18:errorcluster)  [unwired: 2 in, 2 out]
  n90 = for {
    N: w39 -> [_]
    shift-right: [w229] -> w35
    shift-left: "" ("format string") -> [w228]
    tunnel: w36 -> [w219]
    i -> [w227]
    w221 = 2 ("y")
    # "字符从ASCII转成16进制表示"
    n91 = Multiply(x=w227, y=w221) -> (x*y=w220:i32)
    n92 = String Subset(string=w219, offset (0)=w220, length (rest)=w221) -> (substring=w222:string)
    n93 = Hexadecimal String To Number(string=w222) -> (number=w226:u32)  [unwired: 2 in, 1 out]
    n94 = Build Array(w226) -> (w225:u32[])
    n95 = To Unsigned Byte Integer(number=w225) -> (unsigned 8bit integer=w224:u8[])
    n96 = Byte Array To String(unsigned byte array=w224) -> (string=w223:string)
    n97 = Concatenate Strings(w228, w223) -> (w229:string)
  }
  n98 = Merge Errors(w19, w18) -> (→"error out 3":errorcluster)
  n99 = case shown="False" "gps" {
    tunnel: w35 -> [_ w231]
    tunnel: ["\u0000" ("format string") w231] -> w34
    frame False {
    }
    frame True {
    }
  }
  n100 = case shown="0, Default" "coarse counter width" {
    tunnel: [u64 549755812864 ("port") u64 288230376151710720 ("port")] -> w12
    frame 0, Default {
    }
    frame 1 {
    }
  }
  n101 = Increment(x="Counter Setting") -> (x+1=w49:dbl)
  n102 = Divide(x=w53, y="Counter Setting") -> (x/y=w52:dbl)
  n103 = while {
    tunnel: w90 -> [w291]
    tunnel: [w271] -> w61
    tunnel: [w260] -> w83
    shift-right: [w288] -> w65
    shift-left: w10 -> [w289]
    shift-right: [w280] -> _
    shift-left: w60 -> [w287]
    tunnel: "Events" -> [w286]
    shift-right: [w285] -> _
    shift-left: w76 -> [w237]
    shift-right: [w284] -> _
    shift-left: u32 0 ("element") -> [w283]
    shift-right: [w282] -> _
    shift-left: w8 -> [w273]
    shift-right: [w275] -> _
    shift-left: w9 -> [w281]
    tunnel: w14 -> [w267]
    shift-right: [w279] -> _
    shift-left: 0 -> [w254]
    shift-right: [w277] -> _
    shift-left: w31 -> [w276]
    tunnel: w15 -> [_]
    tunnel: w21 -> [w272]
    shift-right: [w268] -> _
    shift-left: w58 -> [w269]
    tunnel: w32 -> [w241]
    tunnel: w53 -> [w265]
    tunnel: w52 -> [w264]
    shift-right: [w259] -> w51
    shift-left: w91 -> [w290]
    tunnel: w49 -> [w258]
    tunnel: w46 -> [w251]
    tunnel: w34 -> [w249]
    tunnel: w31 -> [w248]
    tunnel: "通道数量" -> [w242]
    tunnel: w12 -> [w238]
    shift-right: [w234] -> _
    shift-left: w3 -> [w235]
    tunnel: w2 -> [_]
    tunnel: w1 -> [_]
    stop <- w240 stop-if-true
    n104 = local read "save data"() -> (w253:bool)
    n105 = Dequeue Element(queue=w272) -> (element=w244:string, error out=w271:errorcluster)  [unwired: 2 in, 2 out]
    n106 = case shown="True" w253 {
      tunnel: w291 -> [w304 w312]
      tunnel: w290 -> [w305 w311]
      tunnel: w244 -> [_ w308]
      tunnel: [w305 w307] -> w263
      tunnel: [w304 w306] -> w261
      frame False {
      }
      frame True {
        n107 = Write to Binary File(file (use dialog)=w311, data=w308, error in=w312, 5:FALSE ("prepend array or string size? (T)"), 9:T2."big-endian, network order" ("byte order (0:big-endian, network order)")) -> (refnum out=w307:refnum<file>, error out=w306:errorcluster)  [unwired: 1 in, 1 out]
      }
    }
    n108 = String Length(string=w244) -> (length=w255:i32)
    n109 = case shown="True" TRUE {
      tunnel: w276 -> [w324 w334]
      tunnel: [w324 w335] -> w257
      tunnel: w254 -> [w323 w333]
      tunnel: w255 -> [_ w332]
      tunnel: [w323 w331] -> w256
      tunnel: w251 -> [_ w330]
      tunnel: w248 -> [_ w328]
      tunnel: [FALSE w325] -> w247
      frame False {
      }
      frame True {
        n110 = Get Date/Time In Seconds() -> (seconds since 1Jan1904=w329:timestamp)
        n111 = Subtract(x=w329, y=w334) -> (x-y=w337:dbl)
        n112 = Subtract(x=w329, y=w328) -> (x-y=w327:dbl)
        n113 = Greater Or Equal?(x=w327, y="timeout") -> (x >= y?=w325:bool)
        n114 = Greater Or Equal?(x=w337, y=1.0) -> (x >= y?=w338:bool)
        n115 = case shown="True" w338 {
          tunnel: w337 -> [_ w349]
          tunnel: w329 -> [_ w347]
          tunnel: [w342 w347] -> w335
          tunnel: w334 -> [w342 _]
          tunnel: w333 -> [w341 w344]
          tunnel: w332 -> [w340 _]
          tunnel: [w339 0] -> w331
          tunnel: w330 -> [_ w343]
          frame False {
            n116 = Add(x=w340, y=w341) -> (x+y=w339:i32)
          }
          frame True {
            n117 = Divide(x=w344, y=w343) -> (x/y=w346:dbl)
            n118 = Divide(x=w346, y=w349) -> (x/y=→"rate":dbl)
          }
        }
      }
    }
    n119 = local read "display"() -> (w252:bool)
    n120 = case shown="True" w252 {
      tunnel: w244 -> [_ w303]
      frame False {
      }
      frame True {
        "element" <- w303
      }
    }
    n121 = Unbundle By Name(w271) -> ("status"=w270:bool)
    n122 = case shown="True" "display" {
      tunnel: w273 -> [_ w351]
      tunnel: w237 -> [_ w350]
      frame False {
      }
      frame True {
        "Cal Table" <- w351
        "event" <- w350
      }
    }
    n123 = String Length(string=w244) -> (length=w246:i32)
    n124 = local read "stop"() -> (w239:bool)
    n125 = for {
      N: w246 -> [_]
      tunnel: w244 -> [w300]
      tunnel: [w300] -> w245
      tunnel: [w299] -> w243
      tunnel: w241 -> [w297]
      i -> [w299]
      stop <- w293 stop-if-true
      n126 = Index Array(array=w297) -> (element=w298:string)  [unwired: 1 in]
      n127 = Index Array(array=w297, index=1) -> (element=w295:string)
      n128 = String Subset(string=w300, offset (0)=w299, length (rest)=2 ("length (rest)")) -> (substring=w294:string)
      n129 = Equal?(x=w294, y=w298) -> (x = y?=w301:bool)
      n130 = Equal?(x=w294, y=w295) -> (x = y?=w292:bool)
      n131 = Or(x=w301, y=w292) -> (x .or. y?=w293:bool)
    }
    n132 = case shown="True" "replace dat" {
      tunnel: w263 -> [w314 w320]
      tunnel: [w314 w319] -> w259
      tunnel: w261 -> [w313 w316]
      tunnel: [w313 w315] -> w260
      frame False {
      }
      frame True {
        n133 = Close File(refnum=w320, error in=w316) -> (path=w321:path, error out=w317:errorcluster)
        n134 = Open/Create/Replace File(file path (use dialog)=w321, error in=w317, operation (0:open)=T1."replace or create") -> (refnum out=w319:refnum<file>, error out=w315:errorcluster)  [unwired: 3 in, 1 out]
      }
    }
    n135 = Greater Or Equal?(x=w283, y=w286) -> ()  [unwired: 1 out]
    n136 = Compound Arithmetic op=OR(FALSE ("x"), w270, w247, w239) -> (w240:bool)
    n137 = String Subset(string=w245, offset (0)=w243) -> (substring=w236:string)  [unwired: 1 in]
    n138 = global write "gloabal.vi" "stop"(w240) -> ()
    n139 = while {
      tunnel: w236 -> [w372]
      shift-right: [w442] -> w288
      shift-left: w289 -> [w440]
      shift-right: [w438] -> w280
      shift-left: w287 -> [w439]
      shift-right: [w435] -> w285
      shift-left: w237 -> [w434]
      tunnel: [w433] -> w284
      tunnel: w283 -> [w432]
      shift-right: [w430] -> w282
      shift-left: w273 -> [w431]
      tunnel: w267 -> [w428]
      shift-right: [w427] -> w275
      shift-left: w281 -> [w397]
      shift-right: [w424] -> w268
      shift-left: w269 -> [w425]
      tunnel: w236 -> [w391]
      tunnel: w265 -> [w404]
      tunnel: w264 -> [w403]
      tunnel: w258 -> [w396]
      tunnel: w249 -> [w386]
      tunnel: w242 -> [w374]
      tunnel: w241 -> [w373]
      tunnel: w238 -> [w369]
      tunnel: w236 -> [w359]
      shift-right: [w361] -> w234
      shift-left: w235 -> [w363]
      i -> [w443]
      stop <- w399 stop-if-true
      (unwired) 10 ("length (rest)")
      (unwired) u64 8323072 ("port")
      (unwired) i16 -16 ("y")
      n140 = Multiply(x=w443, y=16 ("length (rest)")) -> (x*y=w364:i32)
      n141 = local read "display"() -> (w426:bool)
      n142 = Add(x=w364, y=8 ("length (rest)")) -> (x+y=w416:i32)
      n143 = Add(x=w364, y=7 ("length (rest)")) -> (x+y=w393:i32)
      n144 = Add(x=w364, y=3 ("length (rest)")) -> (x+y=w366:i32)
      n145 = Add(x=w364, y=0 ("length (rest)")) -> (x+y=w402:i32)
      n146 = String Subset(string=w372, offset (0)=0, length (rest)=2 ("length (rest)")) -> (substring=w375:string)
      "name (unnamed)" <- w375
      n147 = String Subset(string=w372, offset (0)=w402, length (rest)=16 ("y")) -> (substring=w400:string)
      n148 = String Subset(string=w372, offset (0)=w402, length (rest)=8 ("length (rest)")) -> (substring=w384:string)
      n149 = String Subset(string=w391, offset (0)=w416, length (rest)=8 ("length (rest)")) -> (substring=w381:string)
      n150 = String Subset(string=w391, offset (0)=w393, length (rest)=4 ("length (rest)")) -> (substring=w380:string)
      n151 = Search 1D Array(1D array=w373, element=w375) -> (index of element=w376:i32)  [unwired: 1 in]
      n152 = case shown="True" w426 {
        tunnel: w440 -> [_ w489]
        frame False {
        }
        frame True {
          n153 = Index Array(array=w489, index (col)="channel for cal") -> (element=→"cal":i64[])  [unwired: 1 in]
        }
      }
      n154 = String Subset(string=w359, offset (0)=w366, length (rest)=4 ("length (rest)")) -> (substring=w357:string)
      n155 = String Length(string=w400) -> (length=w437:i32)
      n156 = Less?(x=w437, y=16) -> (x < y?=w399:bool)
      n157 = String Subset(string=w384, length (rest)=1 ("length (rest)")) -> (substring=w421:string)  [unwired: 1 in]
      n158 = String Subset(string=w384, offset (0)=7, length (rest)=1 ("length (rest)")) -> (substring=w405:string)
      n159 = Multiply(x=w376, y=w374) -> (x*y=w370:i32)
      n160 = Not Equal?(x="", y=w357) -> (x != y?=w358:bool)
      n161 = String Subset(string=w384, offset (0)=2, length (rest)=1 ("length (rest)")) -> (substring=w382:string)
      n162 = Equal?(x=w421, y="Z" ("format string")) -> (x = y?=w407:bool)
      n163 = Equal?(x=w405, y=w386) -> (x = y?=w406:bool)
      n164 = String To Byte Array(string=w381) -> (unsigned byte array=w413:u8[])
      n165 = String To Byte Array(string=w380) -> (unsigned byte array=w387:u8[])
      n166 = String To Byte Array(string=w382) -> (unsigned byte array=w445:u8[])
      n167 = for {
        shift-right: [w660] -> w410
        shift-left: "" ("format string") -> [w657]
        tunnel: w445 -> [w661] mode=indexing
        n168 = Number To Hexadecimal String(2:w661) -> (0:w653:string)  [unwired: 1 in]
        n169 = String Length(string=w653) -> (length=w659:i32)
        n170 = Equal?(x=w659, y=2) -> (x = y?=w656:bool)
        n171 = Concatenate Strings("0" ("format string"), w653) -> (w655:string)
        n172 = Select(t=w653, s=w656, f=w655) -> (s? t:f=w652:string)
        n173 = Concatenate Strings(w657, w652) -> (w660:string)
      }
      n174 = for {
        shift-right: [w485] -> w411
        shift-left: "" ("format string") -> [w477]
        tunnel: w413 -> [w486] mode=indexing
        n175 = Number To Hexadecimal String(2:w486) -> (0:w479:string)  [unwired: 1 in]
        n176 = String Length(string=w479) -> (length=w484:i32)
        n177 = Concatenate Strings("0" ("format string"), w479) -> (w481:string)
        n178 = Equal?(x=w484, y=2) -> (x = y?=w482:bool)
        n179 = Select(t=w479, s=w482, f=w481) -> (s? t:f=w478:string)
        n180 = Concatenate Strings(w477, w478) -> (w485:string)
      }
      n181 = for {
        shift-right: [w475] -> w390
        shift-left: "" ("format string") -> [w467]
        tunnel: w387 -> [w476] mode=indexing
        n182 = Number To Hexadecimal String(2:w476) -> (0:w469:string)  [unwired: 1 in]
        n183 = String Length(string=w469) -> (length=w474:i32)
        n184 = Concatenate Strings("0" ("format string"), w469) -> (w471:string)
        n185 = Equal?(x=w474, y=2) -> (x = y?=w472:bool)
        n186 = Select(t=w469, s=w472, f=w471) -> (s? t:f=w468:string)
        n187 = Concatenate Strings(w467, w468) -> (w475:string)
      }
      n188 = Not(x=w399) -> (.not. x?=w398:bool)
      n189 = Compound Arithmetic op=AND(w407, w406, w398) -> (w419:bool)
      n190 = Hexadecimal String To Number(string=w410, default (0uL)=u64 0 ("default (0 U32)")) -> (number=w441:u64)  [unwired: 1 in, 1 out]
      n191 = Hexadecimal String To Number(string=w411, default (0uL)=u64 0 ("default (0 U32)")) -> (number=w379:u64)  [unwired: 1 in, 1 out]
      n192 = Hexadecimal String To Number(string=w390, default (0uL)=u64 0 ("default (0 U32)")) -> (number=w368:u64)  [unwired: 1 in, 1 out]
      n193 = And(x=w441, y=u64 127 ("port")) -> (x .and. y?=w371:u64)
      "channel number" <- w371
      n194 = Add(x=w370, y=w371) -> (x+y=w362:u64)
      n195 = case shown="True" w358 {
        tunnel: w363 -> [w447 w453]
        tunnel: w362 -> [_ w451]
        tunnel: [w447 w450] -> w361
        tunnel: w357 -> [_ w449]
        frame False {
        }
        frame True {
          n196 = String To Byte Array(string=w449) -> (unsigned byte array=w454:u8[])
          n197 = for {
            shift-right: [w465] -> w448
            shift-left: "" ("format string") -> [w457]
            tunnel: w454 -> [w466] mode=indexing
            n198 = Number To Hexadecimal String(2:w466) -> (0:w459:string)  [unwired: 1 in]
            n199 = String Length(string=w459) -> (length=w464:i32)
            n200 = Concatenate Strings("0" ("format string"), w459) -> (w461:string)
            n201 = Equal?(x=w464, y=2) -> (x = y?=w462:bool)
            n202 = Select(t=w459, s=w462, f=w461) -> (s? t:f=w458:string)
            n203 = Concatenate Strings(w457, w458) -> (w465:string)
          }
          n204 = Hexadecimal String To Number(string=w448, default (0uL)=u64 0 ("default (0 U32)")) -> (number=w452:u64)  [unwired: 1 in, 1 out]
          n205 = Replace Array Subset(array=w453, new element=w452, index=w451) -> (w450:u32[])
        }
      }
      n206 = case shown="True" w419 {
        tunnel: w379 -> [_ w498]
        tunnel: w432 -> [w493 w513]
        tunnel: w440 -> [w496 w522]
        tunnel: [w496 w521] -> w442
        tunnel: [w495 w518] -> w438
        tunnel: w439 -> [w495 w517]
        tunnel: w362 -> [_ w503]
        tunnel: w434 -> [w494 w516]
        tunnel: [w494 w515] -> w435
        tunnel: [w493 w514] -> w433
        tunnel: w431 -> [w492 w512]
        tunnel: [w492 w511] -> w430
        tunnel: w397 -> [w491 w509]
        tunnel: [w491 w508] -> w427
        tunnel: w428 -> [_ w507]
        tunnel: w425 -> [w490 w505]
        tunnel: [w490 w504] -> w424
        tunnel: w404 -> [_ w502]
        tunnel: w403 -> [_ w501]
        tunnel: w396 -> [_ w500]
        tunnel: w368 -> [_ w499]
        tunnel: w369 -> [_ w497]
        frame False {
          (unwired) FALSE
        }
        frame True {
          n207 = Index Array(array=w512, index=w503) -> (element=w510:u32)
          n208 = Greater?(x=w510, y=w500) -> (0:w506:bool)
          n209 = And(x=w498, y=u64 1023 ("port")) -> (x .and. y?=w519:u64)
          n210 = case shown="False" w506 {
            tunnel: w522 -> [w538 w617]
            tunnel: [w537 w617] -> w521
            tunnel: w519 -> [w529 w575]
            tunnel: [w536 w607] -> w518
            tunnel: w517 -> [w536 w624]
            tunnel: w513 -> [w534 _]
            tunnel: w503 -> [w532 w605]
            tunnel: w516 -> [w535 w623]
            tunnel: [w535 w622] -> w515
            tunnel: [w534 w620] -> w514
            tunnel: w510 -> [w530 _]
            tunnel: w512 -> [w533 w619]
            tunnel: [w531 w619] -> w511
            tunnel: w510 -> [w527 _]
            tunnel: w500 -> [w524 _]
            tunnel: w509 -> [w526 w609]
            tunnel: [w525 w609] -> w508
            tunnel: w507 -> [_ w608]
            tunnel: w505 -> [w523 w602]
            tunnel: [w523 w601] -> w504
            tunnel: w503 -> [_ w598]
            tunnel: w502 -> [_ w596]
            tunnel: w501 -> [_ w597]
            tunnel: w499 -> [_ w591]
            tunnel: w499 -> [_ w580]
            tunnel: w498 -> [_ w574]
            tunnel: w497 -> [_ w572]
            frame False {
              n211 = Equal?(x=w527, y=w524) -> (x = y?=w528:bool)
              n212 = case shown="False" w528 {
                tunnel: w538 -> [w549 w555]
                tunnel: [w547 w555] -> w537
                tunnel: w533 -> [w545 w553]
                tunnel: w532 -> [w544 w550]
                tunnel: [w542 w552] -> w531
                tunnel: w530 -> [w541 w551]
                tunnel: w529 -> [w540 _]
                tunnel: w526 -> [w539 w557]
                tunnel: [w539 w556] -> w525
                frame False {
                  n213 = Index Array(array=w549, index (row)=w540, index (col)=w544) -> (element=w548:i64)
                  n214 = Increment(x=w548) -> (x+1=w546:i64)
                  n215 = Replace Array Subset(array=w549, new element=w546, index (row)=w540, index (col)=w544) -> (w547:i64[][])
                  n216 = Increment(x=w541) -> (x+1=w543:u32)
                  n217 = Replace Array Subset(array=w545, new element=w543, index=w544) -> (w542:u32[])
                  "Calibration Counter" <- w541
                }
                frame True {
                  n218 = for {
                    N: 2048 -> [_]
                    tunnel: w555 -> [w567]
                    tunnel: w550 -> [w560]
                    shift-right: [w562] -> w556
                    shift-left: w557 -> [w563]
                    i -> [w559]
                    n219 = Array Subset(array=w567, index (row)=0 ("索引"), length (row)=w559, index (col)=w560, length (col)=1 ("长度")) -> (w564:i64[][])
                    n220 = Add Array Elements(numeric array=w564) -> (sum=w561:i64)
                    n221 = Replace Array Subset(array=w563, new element=w561, index (row)=w559, index (col)=w560) -> (w562:u32[][])
                  }
                  n222 = Increment(x=w551) -> (x+1=w554:u32)
                  n223 = Replace Array Subset(array=w553, new element=w554, index=w550) -> (w552:u32[])
                }
              }
            }
            frame True {
              (unwired) 0.0 ("x")
              w614 = 0 ("索引 (行)")
              w616 = 1 ("长度")
              # "正式取数"
              n224 = And(x=w580, y=u64 126976 ("port")) -> (x .and. y?=w588:u64)
              n225 = And(x=w591, y=u64 4032 ("port")) -> (x .and. y?=w594:u64)
              n226 = Logical Shift(y=i16 -6, x=w594) -> (x << y=w576:u64)
              n227 = Logical Shift(y=i16 -12, x=w588) -> (x << y=w587:u64)
              n228 = And(x=w580, y=u64 63 ("port")) -> (x .and. y?=w568:u64)
              "x .and. y?" <- w568
              n229 = And(x=w574, y=w572) -> (x .and. y?=w573:u64)
              "fine 4" <- w573
              n230 = Multiply(x=u64 3600, y=w587) -> (x*y=w583:u64)
              n231 = Multiply(x=u64 60, y=w576) -> (x*y=w584:u64)
              n232 = Logical Shift(y=i16 -10, x=w573) -> (x << y=w570:u64)
              "coarse" <- w570
              n233 = Add(x=w584, y=w583) -> (x+y=w582:u64)
              n234 = Add(x=w582, y=w568) -> (x+y=w571:u64)
              "second stamp" <- w571
              n235 = Add(x=w570, y=w571) -> (x+y=w569:u64)
              n236 = Equal?(x=w598, y=u32 2) -> (x = y?=w600:bool)
              n237 = case shown="True" w600 {
                tunnel: w602 -> [w629 w632]
                tunnel: w569 -> [_ w631]
                tunnel: [w629 w630] -> w601
                frame False {
                }
                frame True {
                  n238 = Build Array (concatenate)(w632, w631) -> (w630:u64[])
                }
              }
              "cal 2" <- w601
              n239 = case shown="True" TRUE {
                tunnel: [w639 w647] -> w626
                tunnel: w617 -> [_ _]
                tunnel: w605 -> [w644 w645]
                tunnel: w575 -> [w642 w650]
                tunnel: w609 -> [w643 w651]
                frame False {
                  w638 = 0 ("index (row)")
                  w641 = 1 ("长度")
                  n240 = Decrement(x=w644) -> (x-1=w637:u64)
                  n241 = Array Subset(array=w643, index (row)=w642, length (row)=w641, index (col)=w637, length (col)=w641) -> (w640:u32[][])
                  n242 = Index Array(array=w640, index (row)=w638, index (col)=w638) -> (element=w639:u32)
                }
                frame True {
                  w646 = 0 ("index (row)")
                  w649 = 1 ("长度")
                  n243 = Array Subset(array=w651, index (row)=w650, length (row)=w649, index (col)=w645, length (col)=w649) -> (w648:u32[][])
                  n244 = Index Array(array=w648, index (row)=w646, index (col)=w646) -> (element=w647:u32)
                }
              }
              n245 = Multiply(x=w569, y=w596) -> (x*y=w579:dbl)
              n246 = Index Array(array=w623, index=w605) -> (element=w620:u32)
              n247 = Array Subset(array=w617, index (row)=w575, length (row)=w616, index (col)=w605, length (col)=w616) -> (w615:i64[][])
              n248 = Index Array(array=w615, index (row)=w614, index (col)=w614) -> (element=w613:i64)
              n249 = Divide(x=w613, y=u32 2) -> (x/y=w618:dbl)
              n250 = Increment(x=w620) -> (x+1=w621:u32)
              n251 = Add(x=w626, y=w618) -> (x+y=w625:dbl)
              n252 = Add(x=w579, y=0.0) -> (x+y=w578:dbl)
              n253 = Multiply(x=w625, y=w597) -> (x*y=w611:dbl)
              n254 = Subtract(x=w596, y=w611) -> (x-y=w595:dbl)
              n255 = Add(x=w595, y=w578) -> (x+y=w612:dbl)
              n256 = Replace Array Subset(array=w623, new element=w621, index=w605) -> (w622:u32[])
              n257 = Replace Array Subset(array=w624, new element=w612, index=w605) -> (w606:dbl[])
              n258 = case shown="True" "save data" {
                tunnel: w608 -> [_ w636]
                tunnel: w606 -> [_ w634]
                frame False {
                }
                frame True {
                  n259 = call-poly <vilib>:"Write Delimited Spreadsheet.vi"("file path (dialog if empty)"=w636, "1D data"=w634, "append to file? (new file:F)"="append csv", "delimiter (\\t)"="," ("delimiter (\\t)")) -> ()  [unwired: 10 in, 2 out]
                }
              }
              n260 = Replace Array Subset(array=w606, new element=0.0 ("new element/subarray"), index=w605) -> (w607:dbl[])
              "fine" <- w575
            }
          }
        }
      }
      n261 = Decimate 1D Array(w361) -> (→"pmt trigger rate":u32[])  [unwired: 1 out]
    }
    n262 = case shown="False" "RST" {
      tunnel: w256 -> [w353 _]
      tunnel: [w353 0] -> w279
      tunnel: [w352 w354] -> w277
      tunnel: w257 -> [w352 _]
      frame False {
      }
      frame True {
        n263 = Get Date/Time In Seconds() -> (seconds since 1Jan1904=w354:timestamp)
      }
    }
  }
  "error out 2" <- w61
  n264 = Close File(refnum=w51, error in=w83) -> (error out=→"error out":errorcluster)  [unwired: 1 out]
  n265 = call-poly <vilib>:"Write Delimited Spreadsheet.vi"("file path (dialog if empty)"=w64, "2D data"=w65, "append to file? (new file:F)"=FALSE, "transpose? (no:F)"=TRUE, "delimiter (\\t)"="," ("delimiter (\\t)")) -> ()  [unwired: 9 in, 2 out]
